vi "Process File.vi"(8 "error in (no error)":errorcluster, 10 "File":path, 11 "Integrate in":refnum<class "Integrate.lvclass">) -> (0 "error out":errorcluster, 2 "File out":path, 3 "Integrate out":refnum<class "Integrate.lvclass">)   [LabVIEW 2016, in "Integrate.lvclass"]
uses:
  Integrate.lvclass
  C:/Program Files (x86)/National Instruments/LabVIEW 2016/vi.lib/ActorFramework/Actor/Actor.lvclass
  <vilib>/ActorFramework/Actor/Actor.lvclass/Actor.ctl
  Channel peak.ctl
  Monitor-Pulse Messages/Write Peak Field Msg/Write Peak Field Msg.lvclass/Write Peak Field Msg.ctl
  <vilib>/ActorFramework/Message Enqueuer/Message Enqueuer.lvclass/Message Enqueuer.ctl
  <vilib>/ActorFramework/Message Enqueuer/Enqueue.vi
  Monitor-Pulse Messages/Write Peak Field Msg/Write Peak Field Msg.lvclass
  C:/Program Files (x86)/National Instruments/LabVIEW 2016/vi.lib/ActorFramework/Message/Message.lvclass
  Read Integrate Configuration.vi
  <vilib>/ActorFramework/Message Priority Queue/Priority Enqueue.vi
  <vilib>/ActorFramework/Actor/Actor.lvclass
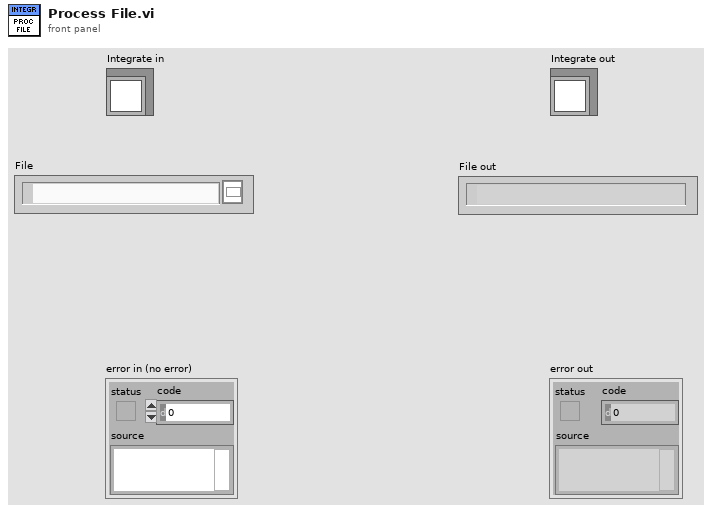
[diagram p1: front panel]
types:
  T1 = typedef "Integrator Configuration.ctl" = cluster{"Integrate":T2[], "Offset duration ":dbl, "TDMS group name":string}
  T2 = typedef "Integrate channel.ctl" = cluster{"Channel":string, "Output name":string, "Factor":dbl, "Start time":dbl, "Duration":dbl, "Fix drift":bool}
  T3 = typedef "Channel peak.ctl" = cluster{"Peak":dbl, "Name":string}
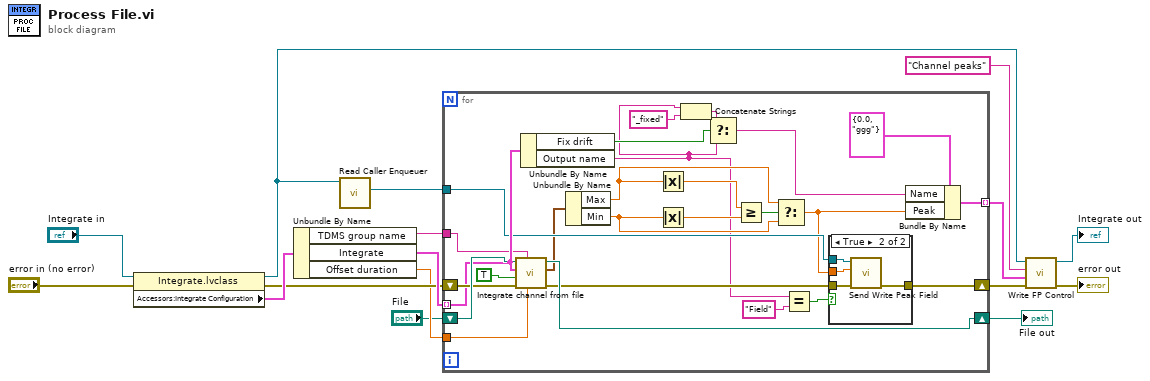
[diagram p0: block diagram]
diagram:
  n1 = property class="Integrate.lvclass"(reference="Integrate in", error in="error in (no error)") -> (reference out=w6:refnum<class "Integrate.lvclass">, error out=w13:errorcluster, "Accessors:Integrate Configuration"=w15:T1)
  n2 = Unbundle By Name(w15) -> ("TDMS group name"=w10:string, "Integrate"=w14:T2[], "Offset duration"=w12:dbl)
  n3 = call <vilib>:"Read Caller Enqueuer.vi"("Actor"=w6) -> ("Caller Enqueuer"=w11:refnum<class "Message Enqueuer.lvclass">)  [unwired: 10 in]
  n4 = for {
    tunnel: w14 -> [w37] mode=indexing
    shift-right: [w41] -> w7
    shift-left: "File" -> [w42]
    tunnel: w12 -> [w38]
    shift-right: [w33] -> w4
    shift-left: w13 -> [w39]
    tunnel: w11 -> [w32]
    tunnel: w10 -> [w31]
    tunnel: [w22] -> w2 mode=indexing
    n5 = call "Integrate channel from file.vi"("Offset duration"=w38, "group name"=w31, "Error In"=w39, "Save data"=TRUE, "Integration settings"=w37, "File Path Control"=w42) -> ("Error Out"=w34:errorcluster, "Min max"=w24:cluster{"Max":dbl, "Min":dbl}, "File Path out"=w41:path)  [unwired: 2 in, 1 out]
    n6 = Unbundle By Name(w37) -> ("Fix drift"=w21:bool, "Output name"=w18:string)
    n7 = Unbundle By Name(w24) -> ("Max"=w26:dbl, "Min"=w29:dbl)
    n8 = Absolute Value(x=w26) -> (abs(x)=w27:dbl)
    n9 = Absolute Value(x=w29) -> (abs(x)=w28:dbl)
    n10 = Concatenate Strings(w18, "_fixed" ("string")) -> (w17:string)
    n11 = Select(t=w17, s=w21, f=w18) -> (s? t:f=w20:string)
    n12 = Greater Or Equal?(x=w27, y=w28) -> (x >= y?=w25:bool)
    n13 = Select(t=w26, s=w25, f=w29) -> (s? t:f=w23:dbl)
    n14 = Equal?(x=w18, y="Field") -> (x = y?=w35:bool)
    n15 = case shown="True" w35 {
      tunnel: w34 -> [w43 w47]
      tunnel: [w43 w46] -> w33
      tunnel: w32 -> [_ w45]
      tunnel: w23 -> [_ w44]
      frame False {
      }
      frame True {
        n16 = call "Send Write Peak Field.vi"("error in (no error)"=w47, "Peak Field"=w44, "Message Enqueuer"=w45) -> ("error out"=w46:errorcluster)  [unwired: 7 in, 1 out]
      }
    }
    n17 = Bundle By Name(cluster=T3 {"Peak"=0.0, "Name"="ggg"} ("Channel peak"), "Name"=w20, "Peak"=w23) -> (w22:T3)
  }
  "File out" <- w7
  n18 = call-dynamic "Write FP Control.vi"("error in (no error)"=w4, "Control Value"=w2, "Control Name"="Channel peaks", "Measure Object in"=w6) -> ("error out"=→"error out":errorcluster, "Measure Object out"=→"Integrate out":refnum<class "Integrate.lvclass">)  [unwired: 6 in]
